vi "Set NodeIDs.vi"(8 "error in (no error)":errorcluster, 9 "Deliminated Char":string=".", 10 "Folder names":string[](array[string]), 11 "Control Refs":refnum<vi>[](array[refnum])) -> (0 "error out":errorcluster, 3 "NodeIDs":string[][](array[string]))   [LabVIEW 2021, in "OPCUA.lvlib"]
uses:
  OPCUA.lvlib
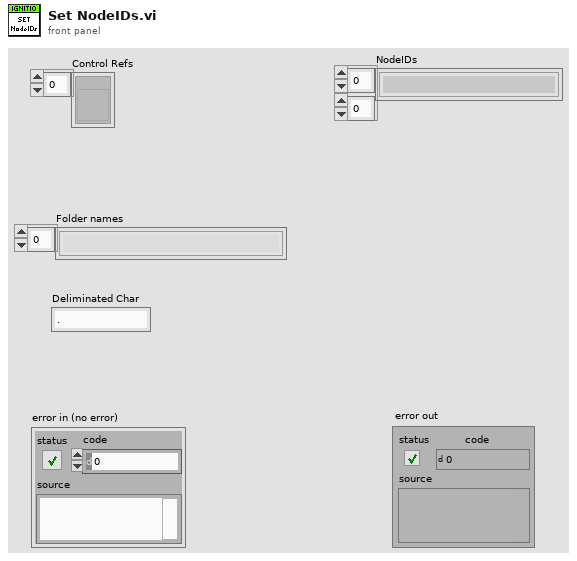
[diagram p1: front panel]
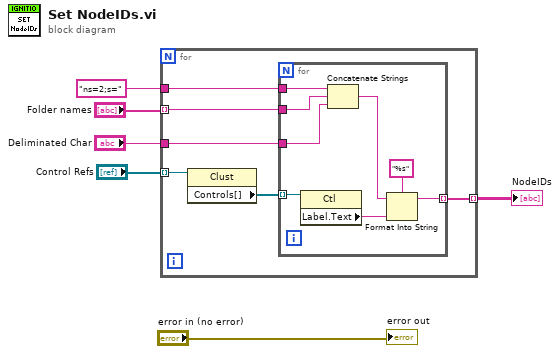
[diagram p0: block diagram]
diagram:
  n1 = for {
    tunnel: "ns=2;s=" ("format string") -> [w12]
    tunnel: [w11] -> w2 mode=indexing
    tunnel: "Folder names" -> [w10] mode=indexing
    tunnel: "Control Refs" -> [w8] mode=indexing
    tunnel: "Deliminated Char" -> [w7]
    n2 = property class="Clust"(reference=w8) -> ("Controls[]"=w9:refnum<vi>[])  [unwired: 1 in, 2 out]
    n3 = for {
      tunnel: w9 -> [w20] mode=indexing
      tunnel: w10 -> [w17]
      tunnel: [w18] -> w11 mode=indexing
      tunnel: w12 -> [w16]
      tunnel: w7 -> [w14]
      n4 = property class="Ctl"(reference=w20) -> ("Label.Text"=w13:string)  [unwired: 1 in, 2 out]
      n5 = Concatenate Strings(w16, w17, w14) -> (w15:string)
      n6 = Format Into String(format string="%s", initial string=w15, w13) -> (resulting string=w18:string)  [unwired: 1 in, 1 out]
    }
  }
  "NodeIDs" <- w2
  "error out" <- "error in (no error)"
